vi "Close Serial Port.vi"(1 "error in (no error)":errorcluster, 2 "Serial Port":refnum<visa-resource-name>="COM1") -> (0 "error out":errorcluster)   [LabVIEW 2017]
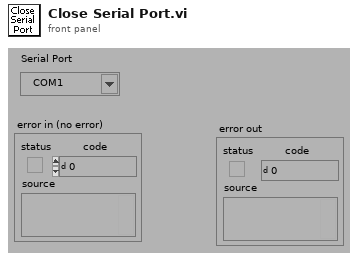
[diagram p1: front panel]
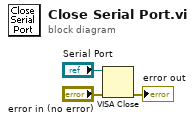
[diagram p0: block diagram]
diagram:
  n1 = VISA Close(VISA resource name="Serial Port", error in (no error)="error in (no error)") -> (error out=→"error out":errorcluster)
